vi "Process.vi"(8 "error in":errorcluster, 11 "SMO.UI.ByRefWithEvents":refnum<class "SMO.UI.ByRefWithEvents.lvclass">) -> (0 "error out":errorcluster, 3 "SMO.UI.ByRefWithEvents out":refnum<class "SMO.UI.ByRefWithEvents.lvclass">)   [LabVIEW 2013, in "SMO.UI.ByRefWithEvents.lvclass"]
doc: "---------------------------------------------------------------\nJKI State Machine Objects™\nhttp://jki.net/state-machine-objects/\nCopyright (C) 2005-2015, JKI <info@jki.net>\nALL RIGHTS RESERVEDJKI State Machine Objects (SMO) 1.0.0.5\nJKI - JKI\nCopyright (c) 2016, JKI"
uses:
  SMO.UI.ByRefWithEvents.lvclass
  <vilib>/JKI/JKI SMO/SMO/Typedefs/Parent Call--Enum.ctl
  <vilib>/JKI/JKI SMO/SMO.UI/SMO.UI.lvclass
  <vilib>/JKI/JKI SMO/SMO/SMO.lvclass
panel:
  out "Data":string
  # "For instructions on how to use the JKI State Machine Objects, examples and video tutorials, visit:\nhttp://jki.net/state-machine-objects/\n\nJKI State Machine Objects™\nhttp://jki.net/state-machine-objects/\nCopyright (C) 2005-2015, JKI <info@jki.net>\nALL RIGHTS RESERVED"
  # "SMO UI Template"
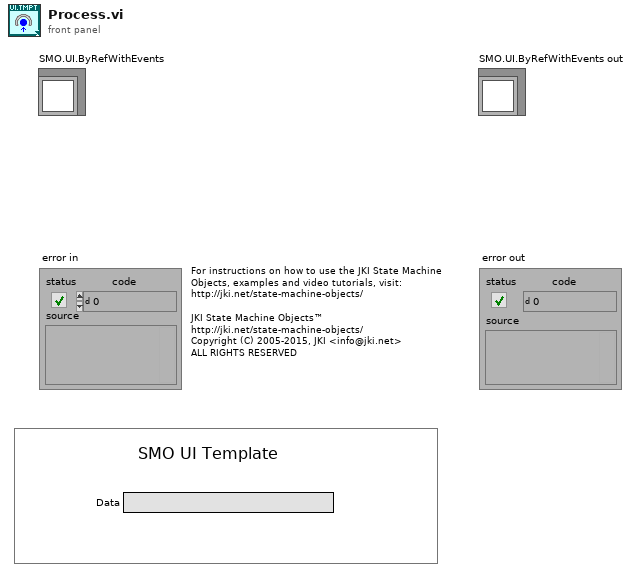
[diagram p1: front panel]
types:
  T1 = typedef "SMO.lvclass/Parent Call--Enum.ctl" = enum16{"Allows parent to run", "Does not request parent to run"}
  T2 = enum32{"invalid app kind", "Development System", "Run Time System", "Student Edition", "Embedded LabVIEW", "Evaluation", "Custom"}
  T3 = enum32{"Invalid", "Standard", "Closed", "Hidden", "Minimized", "Maximized"}
  T4 = cluster{"Core":cluster{"Current VI Reference":refnum<vi>, "Close Panel on Exit?":bool, "error":errorcluster}, "Self Reference":refnum<class "SMO.UI.ByRefWithEvents.lvclass">, "Your string data":string}
  T5 = cluster{"Current VI Reference":refnum<vi>, "Close Panel on Exit?":bool, "error":errorcluster}
  T6 = typedef "SMO.lvclass/Protected Events.ctl" = cluster{"StopProcesses":refnum<user-event>, "AbortProcesses":refnum<user-event>, "Config Changed":refnum<user-event>}
  T7 = typedef "SMO.UI.ByRefWithEvents.lvclass/ProtectedEvents--Cluster.ctl" = cluster{"API_Template":refnum<user-event>}
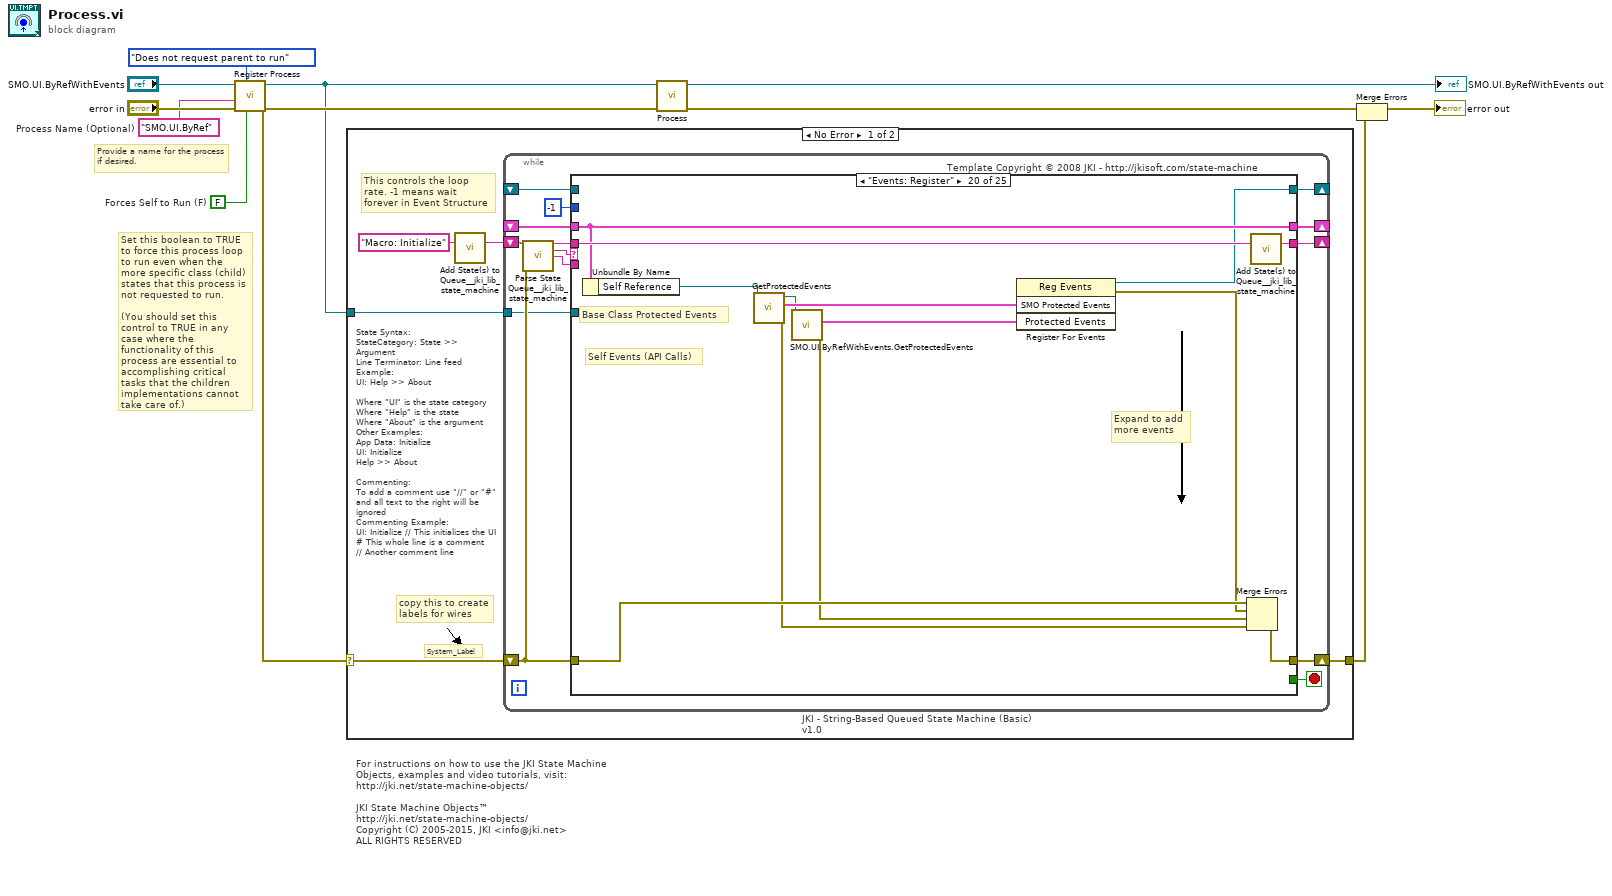
[diagram p0: block diagram]
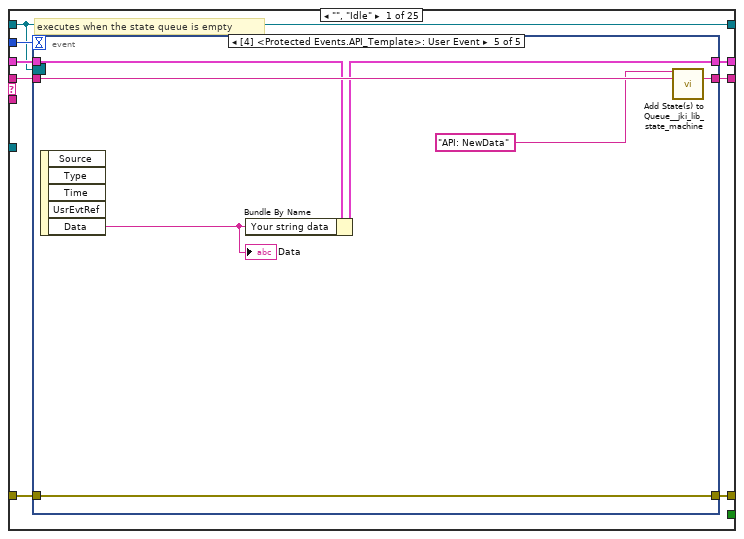
[diagram p2: hidden frame]
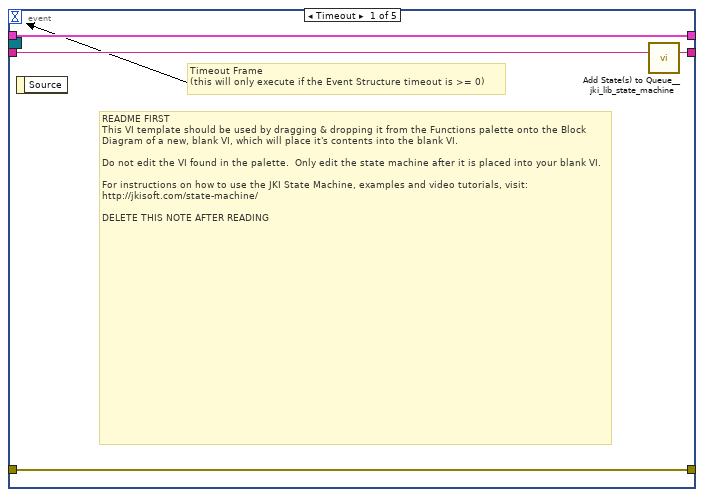
[diagram p3: hidden frame]
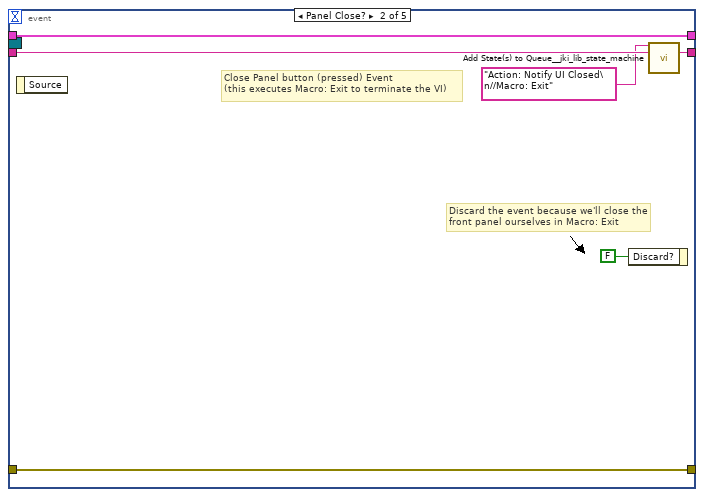
[diagram p4: hidden frame]
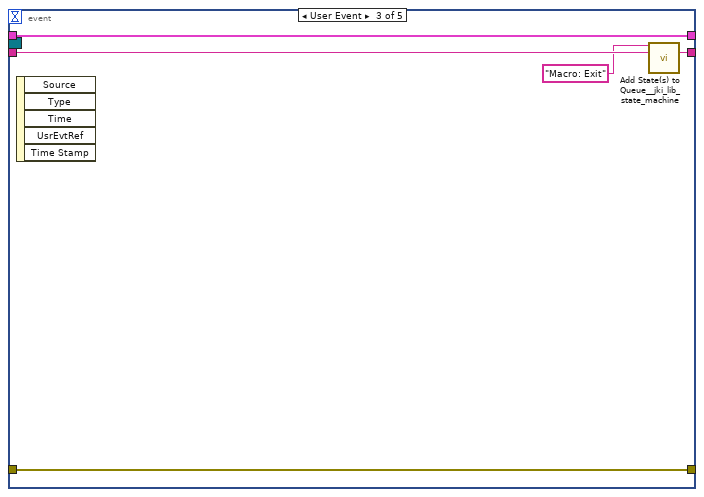
[diagram p5: hidden frame]
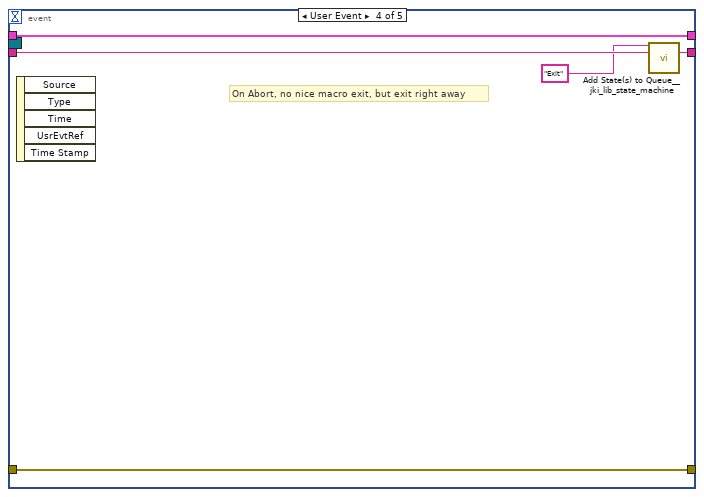
[diagram p6: hidden frame]
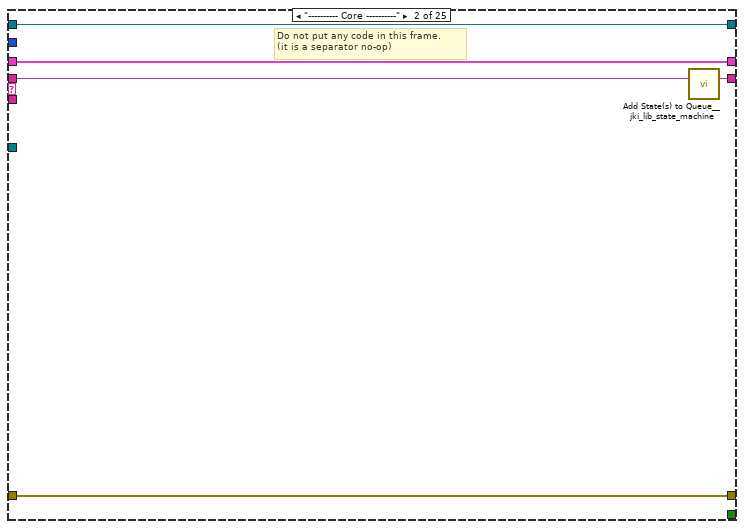
[diagram p7: hidden frame]
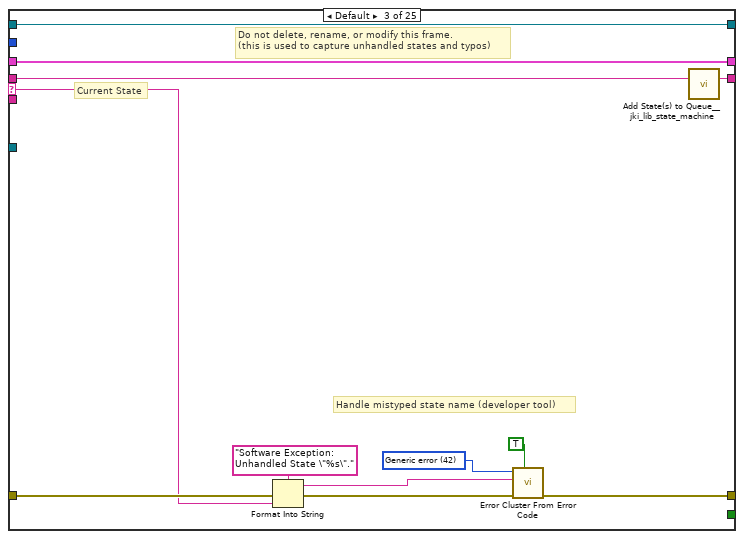
[diagram p8: hidden frame]
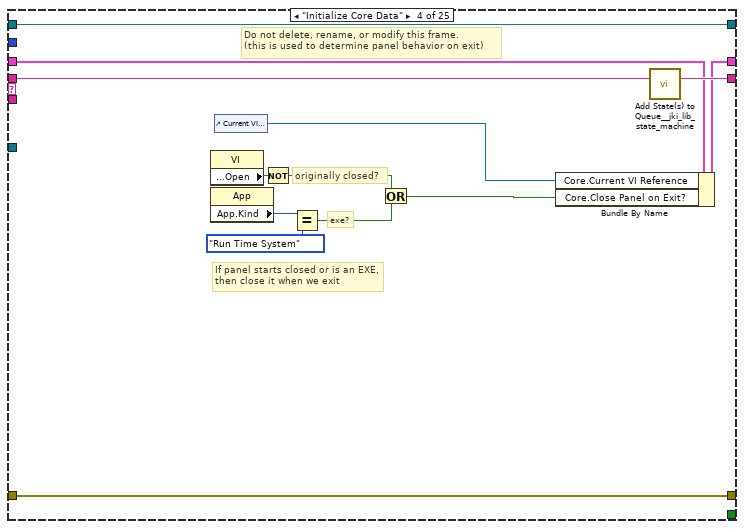
[diagram p9: hidden frame]
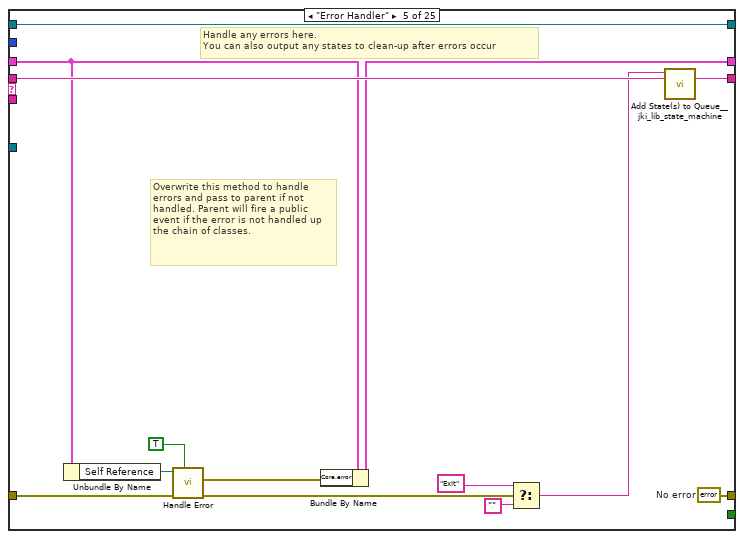
[diagram p10: hidden frame]
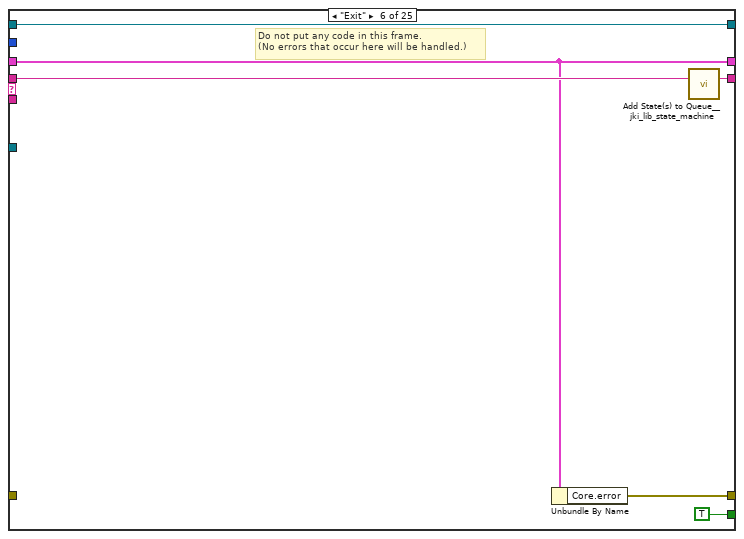
[diagram p11: hidden frame]
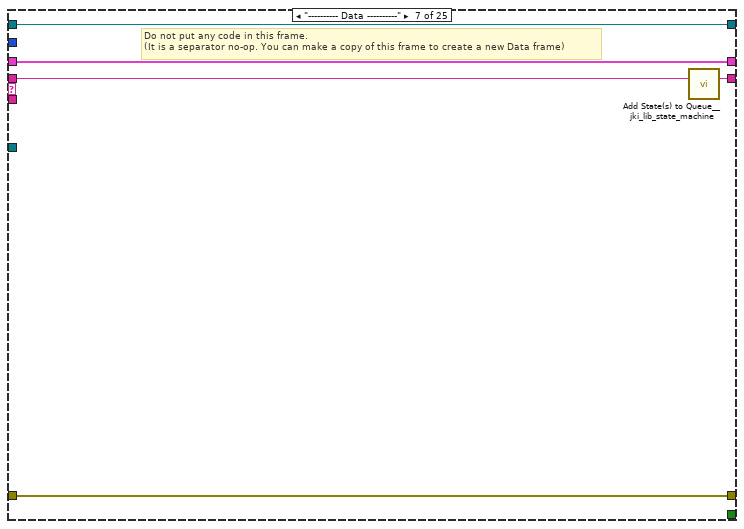
[diagram p12: hidden frame]
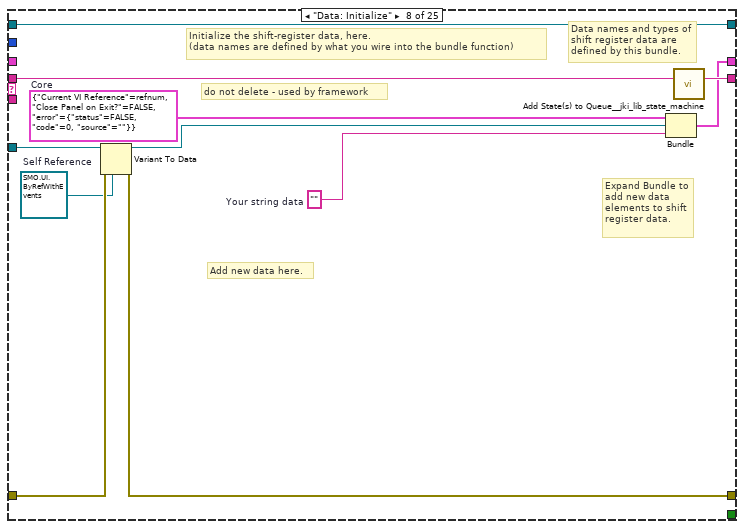
[diagram p13: hidden frame]
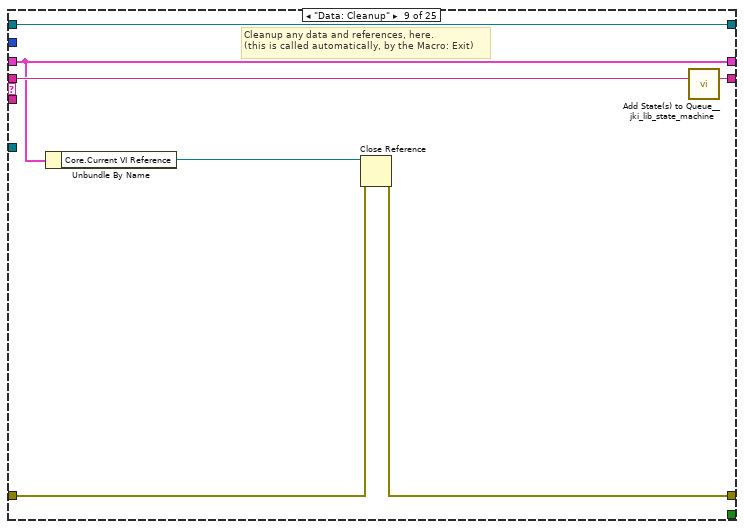
[diagram p14: hidden frame]
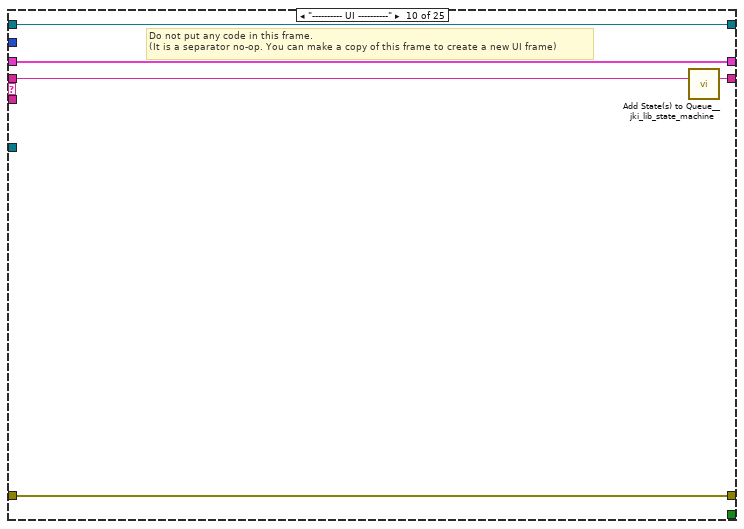
[diagram p15: hidden frame]
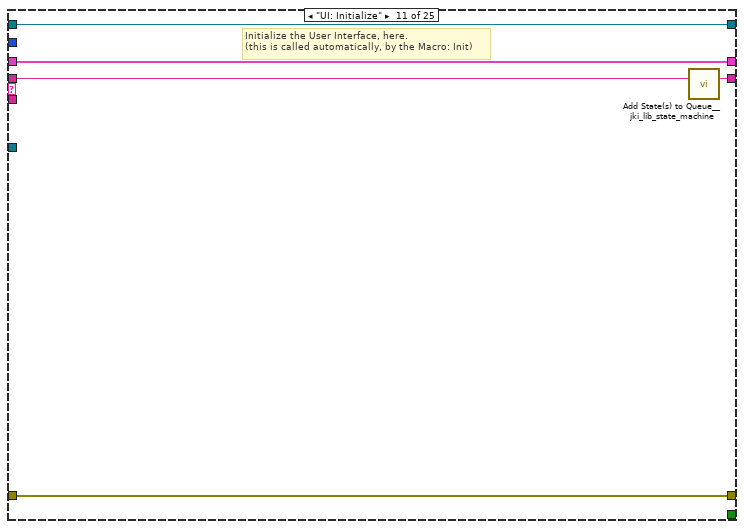
[diagram p16: hidden frame]
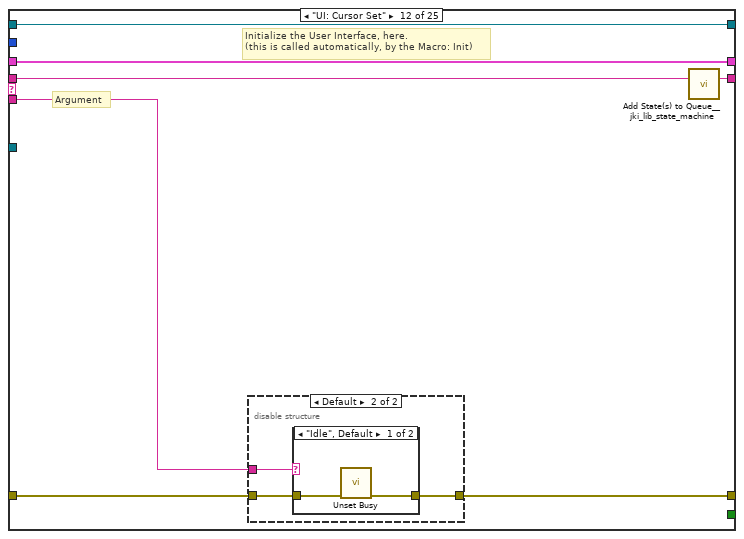
[diagram p17: hidden frame]
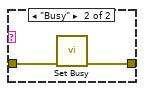
[diagram p19: hidden frame]
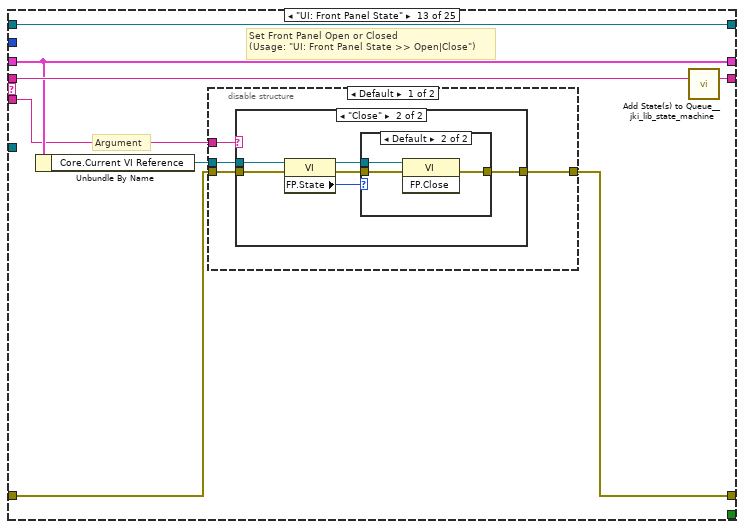
[diagram p20: hidden frame]
diagram:
  w2 = FALSE  # Forces Self to Run (F)
  w1 = "SMO.UI.ByRef"  # Process Name (Optional)
  # "Provide a name for the process\nif desired."
  # "Set this boolean to TRUE to force this process loop to run even when the more specific class (child) states that this process is not requested to run.\n\n(You should set this control to TRUE in any case where the functionality of this process are essential to accomplishing critical tasks that the children implementations cannot take care of.)"
  # "For instructions on how to use the JKI State Machine Objects, examples and video tutorials, visit:\nhttp://jki.net/state-machine-objects/\n\nJKI State Machine Objects™\nhttp://jki.net/state-machine-objects/\nCopyright (C) 2005-2015, JKI <info@jki.net>\nALL RIGHTS RESERVED"
  n1 = call <vilib>:"Register Process.vi"("Forces Self to Run (F)"=w2, "Parent Call"=Parent_Call--Enum."Does not request parent to run", "error in (no error)"="error in", "Process Name (optional)"=w1, "SMO"="SMO.UI.ByRefWithEvents") -> ("error out"=w8:errorcluster, "SMO out"=w7:refnum<class "SMO.UI.ByRefWithEvents.lvclass">)  [unwired: 5 in]
  n2 = case shown="No Error" w8 {
    selector: w8 -> [w13 w292]
    tunnel: w7 -> [w14 _]
    tunnel: [w12 w292] -> w4
    frame No Error {
      # "State Syntax:\nStateCategory: State >> Argument\nLine Terminator: Line feed\nExample:\nUI: Help >> About\n\nWhere \"UI\" is the state category\nWhere \"Help\" is the state\nWhere \"About\" is the argument\nOther Examples:\nApp Data: Initialize\nUI: Initialize\nHelp >> About\n\nCommenting:\nTo add a comment use \"//\" or \"#\" and all text to the right will be ignored\nCommenting Example:\nUI: Initialize // This initializes the UI\n# This whole line is a comment\n// Another comment line"
      # "copy this to create labels for wires"
      # "This controls the loop rate. -1 means wait forever in Event Structure"
      # "System_Label"
      n3 = call <vilib>:"Add State(s) to Queue__jki_lib_state_machine.vi"("State(s) in (\"\")"="Macro: Initialize") -> ("States Out"=w16:string)  [unwired: 14 in]
      n4 = while "JKI - String-Based Queued State Machine (Basic) v1.0" {
        shift-right: [w23] -> _
        shift-left: _ -> [w22]
        shift-right: [w26] -> w12
        shift-left: w13 -> [w20]
        shift-right: [w25] -> _
        shift-left: w16 -> [w27]
        tunnel: w14 -> [w19]
        shift-right: [w18] -> _
        shift-left: _ -> [w17]
        stop <- w24 stop-if-true
        # "Template Copyright © 2008 JKI - http://jkisoft.com/state-machine"
        n5 = call <vilib>:"Parse State Queue__jki_lib_state_machine.vi"("State Queue"=w27, "Error In (no error)"=w20) -> ("Remaining States"=w29:string, "Current State"=w30:string, "Arguments"=w28:string)  [unwired: 11 in]
        n6 = case shown="\"Events: Register\"" w30 {
          selector: w30 -> [_ _ w72 _ _ _ _ _ _ _ _ _ _ _ _ _ _ _ _ _ _ _ _ _ _]
          tunnel: w29 -> [w38 w70 w76 w95 w109 w115 w120 w131 w138 w143 w148 w155 w171 w203 w212 w226 w231 w242 w247 w260 w266 w271 w279 w284 w291]
          tunnel: w28 -> [_ _ _ _ _ _ _ _ _ _ _ w149 w165 _ _ _ _ _ _ _ _ _ _ _ _]
          tunnel: w22 -> [w36 w67 w74 w86 w98 w111 w117 _ w133 w140 w146 w153 w167 w200 w208 w217 w228 w239 w244 w258 w264 w269 w276 w282 w287]
          tunnel: [w35 w68 w78 w92 w100 w110 w118 w126 w134 w141 w145 w150 w168 w201 w210 w224 w229 w233 w245 w250 w262 w267 w273 w280 w285] -> w26
          tunnel: w20 -> [w34 w68 w77 w92 w105 _ w118 w127 w135 w141 w145 w151 w169 w201 w210 w224 w229 w234 w245 w252 w262 w267 w274 w280 w286]
          tunnel: [w37 w69 w75 w94 w108 w114 w119 w130 w137 w142 w147 w154 w170 w202 w211 w225 w230 w241 w246 w259 w265 w270 w278 w283 w290] -> w25
          tunnel: [_ _ _ _ _ TRUE _ _ _ _ _ _ _ _ _ _ _ _ _ _ _ _ _ _ _] -> w24
          tunnel: [w33 w67 w74 w93 w97 w111 w117 w129 w133 w140 w146 w153 w167 w200 w208 w217 w228 w239 w244 w258 w264 w269 w276 w282 w287] -> w23
          tunnel: -1 ("Timeout") -> [w32 _ _ _ _ _ _ _ _ _ _ _ _ _ _ _ _ _ _ _ _ _ _ _ _]
          tunnel: w19 -> [_ _ _ _ _ _ _ w124 _ _ _ _ _ _ _ _ _ _ _ _ _ _ _ _ _]
          tunnel: [w31 w66 w71 w83 w107 w112 w116 w122 w132 w139 w144 w152 w164 w199 w209 w218 w227 w240 w243 w257 w263 w268 w277 w281 w289] -> w18
          tunnel: w17 -> [w31 w66 w71 w83 w107 w112 w116 w122 w132 w139 w144 w152 w164 w199 w209 w218 w227 w240 w243 _ w263 w268 w277 w281 w289]
          frame "", "Idle" {
            # "executes when the state queue is empty"
            n7 = event shown="[4] <Protected Events.API_Template>: User Event" {
              selector: w31 -> [_ _ _ _ _]
              dyn-events: _ -> [_ _ _ _ _]
              timeout: w32 -> [_ _ _ _ _]
              tunnel: w38 -> [w42 w48 w53 w58 w65]
              tunnel: [w41 w47 w52 w57 w64] -> w37
              tunnel: w36 -> [w39 w44 w50 w55 w62]
              tunnel: [w40 w43 w51 w56 w63] -> w35
              tunnel: w34 -> [w40 w43 w51 w56 w63]
              tunnel: [w39 w44 w50 w55 w61] -> w33
              event Timeout {
                # "README FIRST\nThis VI template should be used by dragging & dropping it from the Functions palette onto the Block Diagram of a new, blank VI, which will place it's contents into the blank VI.\n\nDo not edit the VI found in the palette.  Only edit the state machine after it is placed into your blank VI.\n\nFor instructions on how to use the JKI State Machine, examples and video tutorials, visit:\nhttp://jkisoft.com/state-machine/\n\nDELETE THIS NOTE AFTER READING"
                # "Timeout Frame\n(this will only execute if the Event Structure timeout is >= 0)"
                n8 = event-data() -> ()  [unwired: 1 in, 1 out]
                n9 = call <vilib>:"Add State(s) to Queue__jki_lib_state_machine.vi"("State(s) in (\"\")"=w42) -> ("States Out"=w41:string)  [unwired: 14 in]
              }
              event Panel Close? {
                # "Discard the event because we'll close the front panel ourselves in Macro: Exit"
                # "Close Panel button (pressed) Event\n(this executes Macro: Exit to terminate the VI)"
                n10 = event-data() -> ()  [unwired: 1 in, 1 out]
                n11 = event-data("Discard?"=FALSE) -> ()  [unwired: 1 in, 1 out]
                n12 = call <vilib>:"Add State(s) to Queue__jki_lib_state_machine.vi"("State(s) in Front (\"\")"="Action: Notify UI Closed\n//Macro: Exit", "State(s) in (\"\")"=w48) -> ("States Out"=w47:string)  [unwired: 13 in]
              }
              event User Event {
                n13 = event-data() -> ()  [unwired: 1 in, 5 out]
                n14 = call <vilib>:"Add State(s) to Queue__jki_lib_state_machine.vi"("State(s) in Front (\"\")"="Macro: Exit", "State(s) in (\"\")"=w53) -> ("States Out"=w52:string)  [unwired: 13 in]
              }
              event User Event {
                # "On Abort, no nice macro exit, but exit right away"
                n15 = event-data() -> ()  [unwired: 1 in, 5 out]
                n16 = call <vilib>:"Add State(s) to Queue__jki_lib_state_machine.vi"("State(s) in Front (\"\")"="Exit", "State(s) in (\"\")"=w58) -> ("States Out"=w57:string)  [unwired: 13 in]
              }
              event User Event {
                n17 = event-data() -> ("Data"=w59:string)  [unwired: 1 in, 4 out]
                "Data" <- w59
                n18 = Bundle By Name(cluster=w62, "Your string data"=w59) -> (w61:T4)
                n19 = call <vilib>:"Add State(s) to Queue__jki_lib_state_machine.vi"("State(s) in Front (\"\")"="API: NewData", "State(s) in (\"\")"=w65) -> ("States Out"=w64:string)  [unwired: 13 in]
              }
            }
          }
          frame "---------- Core ----------" {
            # "Do not put any code in this frame.\n(it is a separator no-op)"
            n20 = call <vilib>:"Add State(s) to Queue__jki_lib_state_machine.vi"("State(s) in (\"\")"=w70) -> ("States Out"=w69:string)  [unwired: 14 in]
          }
          frame Default {
            w81 = 42 items=["No error", "Argument error", "Memory is full", "Out of zone", "End of file", "File already open", "Generic file I/O error", "File not found", "File permission error", "Disk is full", "Duplicate path", "Too many files open", "System feature not enabled", "Resource file not found", "Cannot add resource", "Resource not found", "Image not found", "Image memory error", "Pen does not exist", "Config type invalid", "Config token not found", "Config parse error", "Config memory error", "Bad external code format", "Bad external code offset", "External code not present", "Null window", "Destroy window error", "Null menu", "Print aborted", "Bad print record", "Print driver error", "Windows error during printing", "Memory error during printing", "Print dialog error", "Generic print error", "Invalid device refnum", "Device not found", "Device parameter error", "Device unit error", "Cannot open device", "Device call aborted", "Generic error", "Cancelled by user", "Object ID too low", "Object ID too high", "Object not in heap", "Unknown heap", "Unknown object (invalid DefProc)", "Unknown object (DefProc not in table)", "Message out of range", "Invalid (null) method", "Unknown message", "Manager call not supported", "Bad address", "Network operation in progress", "Network operation timed out", "Connection is busy", "Network attribute not supported", "Network error", "Address in use", "System out of memory", "Connection aborted", "Connection refused", "Not connected", "Already connected", "Connection closed", "Initialization error (interapplication manager)", "Bad occurrence", "Wait on unbound occurrence handler", "Occurrence queue overflow", "Datalog type conflict", "Unused", "Unrecognized type (interapplication manager)", "Memory corrupt", "Failed to make temporary DLL", "Old CIN version", "Drag socket not found", "Failed to load drop-object", "Failed to register OLE object", "Failed to release OLE object", "Format specifier type mismatch", "Unknown format specifier", "Too few format specifiers", "Too many format specifiers", "Scan failed", "Newer CIN version", "Error converting to variant", "Runtime menu error", "Password tampered", "Variant attribute not found", "Incompatible variant data type", "Event data is not available", "Event Store is not present", "Occurrence is not found", "Event Queue is not created", "Event info is not available", "Refnum passed is NULL", "Error retrieving Class GUID", "Error retrieving CoClass GUID", "Error retrieving TypeLib GUID.", "Bad built application magic bytes.", "Specific driver is different from the specific driver associated with the Logical Name.", "There is no session opened to the class driver.", "Max Error", "MAX - Error with config objects", "MAX - Error loading configuration", "MAX - Group not supported"]
            # "Current State"
            # "Do not delete, rename, or modify this frame.\n(this is used to capture unhandled states and typos)"
            # "Handle mistyped state name (developer tool)"
            n21 = Format Into String(format string="Software Exception: Unhandled State \"%s\"." ("message"), error in=w77, w72) -> (resulting string=w80:string, error out=w79:errorcluster)  [unwired: 1 in]
            n22 = call <vilib>:"Error Cluster From Error Code.vi"("show call chain? (False)"=TRUE, "error in (no error)"=w79, "error message (\"\")"=w80, "error code (0)"=w81) -> ("error out"=w78:errorcluster)  [unwired: 5 in]
            n23 = call <vilib>:"Add State(s) to Queue__jki_lib_state_machine.vi"("State(s) in (\"\")"=w76) -> ("States Out"=w75:string)  [unwired: 14 in]
          }
          frame "Initialize Core Data" {
            # "Do not delete, rename, or modify this frame.\n(this is used to determine panel behavior on exit)"
            # "originally closed?"
            # "exe?"
            # "If panel starts closed or is an EXE, then close it when we exit"
            n24 = property class="VI"() -> ("Front Panel.Open"=w91:bool)  [unwired: 2 in, 2 out]
            n25 = property class="App"() -> ("App.Kind"=w90:T2)  [unwired: 2 in, 2 out]
            n26 = control-ref of="Current VI Reference"() -> (w84:refnum<vi>)
            n27 = Not(x=w91) -> (.not. x?=w88:bool)
            n28 = Equal?(x=w90, y=T2."Run Time System" ("Application:Kind")) -> (x = y?=w87:bool)
            n29 = Or(x=w88, y=w87) -> (x .or. y?=w85:bool)
            n30 = Bundle By Name(cluster=w86, "Core.Current VI Reference"=w84, "Core.Close Panel on Exit?"=w85) -> (w93:T4)
            n31 = call <vilib>:"Add State(s) to Queue__jki_lib_state_machine.vi"("State(s) in (\"\")"=w95) -> ("States Out"=w94:string)  [unwired: 14 in]
          }
          frame "Error Handler" {
            w100 = errorcluster {"status"=FALSE, "code"=0, "source"=""}  # No error
            # "Overwrite this method to handle errors and pass to parent if not handled. Parent will fire a public event if the error is not handled up the chain of classes."
            # "Handle any errors here.\nYou can also output any states to clean-up after errors occur"
            n32 = Unbundle By Name(w98) -> ("Self Reference"=w106:refnum<class "SMO.UI.ByRefWithEvents.lvclass">)
            n33 = call-dynamic "Handle Error.vi"("Stop on Unhandled Error (T)"=TRUE, "error in"=w105, "SMO"=w106) -> ("handling error"=w101:errorcluster, "Unhandled error"=w99:errorcluster)  [unwired: 6 in, 1 out]
            n34 = Bundle By Name(cluster=w98, "Core.error"=w99) -> (w97:T4)
            n35 = Select(t="Exit", s=w101, f="") -> (s? t:f=w102:string)
            n36 = call <vilib>:"Add State(s) to Queue__jki_lib_state_machine.vi"("State(s) in Front (\"\")"=w102, "State(s) in (\"\")"=w109) -> ("States Out"=w108:string)  [unwired: 13 in]
          }
          frame "Exit" {
            # "Do not put any code in this frame.\n(No errors that occur here will be handled.)"
            n37 = Unbundle By Name(w111) -> ("Core.error"=w110:errorcluster)
            n38 = call <vilib>:"Add State(s) to Queue__jki_lib_state_machine.vi"("State(s) in (\"\")"=w115) -> ("States Out"=w114:string)  [unwired: 14 in]
          }
          frame "---------- Data ----------" {
            # "Do not put any code in this frame.\n(It is a separator no-op. You can make a copy of this frame to create a new Data frame)"
            n39 = call <vilib>:"Add State(s) to Queue__jki_lib_state_machine.vi"("State(s) in (\"\")"=w120) -> ("States Out"=w119:string)  [unwired: 14 in]
          }
          frame "Data: Initialize" {
            w121 = T5 {"Current VI Reference"=refnum, "Close Panel on Exit?"=FALSE, "error"={"status"=FALSE, "code"=0, "source"=""}}  # Core
            w125 = refnum<class "SMO.UI.ByRefWithEvents.lvclass"> refnum  # Self Reference
            w128 = ""  # Your string data
            # "do not delete - used by framework"
            # "Expand Bundle to add new data elements to shift register data."
            # "Add new data here."
            # "Data names and types of shift register data are defined by this bundle."
            # "Initialize the shift-register data, here.\n(data names are defined by what you wire into the bundle function)"
            n40 = Variant To Data(error in=w127, type=w125, Variant=w124) -> (data=w123:refnum<class "SMO.UI.ByRefWithEvents.lvclass">, error out=w126:errorcluster)
            n41 = Bundle("Core"=w121, "Self Reference"=w123, "Your string data"=w128) -> (w129:T4)  [unwired: 1 in]
            n42 = call <vilib>:"Add State(s) to Queue__jki_lib_state_machine.vi"("State(s) in (\"\")"=w131) -> ("States Out"=w130:string)  [unwired: 14 in]
          }
          frame "Data: Cleanup" {
            # "Cleanup any data and references, here.\n(this is called automatically, by the Macro: Exit)"
            n43 = Unbundle By Name(w133) -> ("Core.Current VI Reference"=w136:refnum<vi>)
            n44 = Close Reference(reference=w136, error in (no error)=w135) -> (error out=w134:errorcluster)
            n45 = call <vilib>:"Add State(s) to Queue__jki_lib_state_machine.vi"("State(s) in (\"\")"=w138) -> ("States Out"=w137:string)  [unwired: 14 in]
          }
          frame "---------- UI ----------" {
            # "Do not put any code in this frame.\n(It is a separator no-op. You can make a copy of this frame to create a new UI frame)"
            n46 = call <vilib>:"Add State(s) to Queue__jki_lib_state_machine.vi"("State(s) in (\"\")"=w143) -> ("States Out"=w142:string)  [unwired: 14 in]
          }
          frame "UI: Initialize" {
            # "Initialize the User Interface, here.\n(this is called automatically, by the Macro: Init)"
            n47 = call <vilib>:"Add State(s) to Queue__jki_lib_state_machine.vi"("State(s) in (\"\")"=w148) -> ("States Out"=w147:string)  [unwired: 14 in]
          }
          frame "UI: Cursor Set" {
            # "Argument"
            # "Initialize the User Interface, here.\n(this is called automatically, by the Macro: Init)"
            n48 = disable-structure shown="Default" {
              disable-tunnel: w151 -> [w156 w159]
              disable-tunnel: [w156 w158] -> w150
              disable-tunnel: w149 -> [_ w157]
              frame condition #0 {
              }
              frame condition #1 (active) {
                n49 = case shown="\"Idle\", Default" w157 {
                  tunnel: w159 -> [w161 w163]
                  tunnel: [w160 w162] -> w158
                  frame "Idle", Default {
                    n50 = call <vilib>:"Unset Busy.vi"("error in (no error)"=w161) -> ("error out"=w160:errorcluster)  [unwired: 10 in]
                  }
                  frame "Busy" {
                    n51 = call <vilib>:"Set Busy.vi"("error in (no error)"=w163) -> ("error out"=w162:errorcluster)  [unwired: 9 in, 1 out]
                  }
                }
              }
            }
            n52 = call <vilib>:"Add State(s) to Queue__jki_lib_state_machine.vi"("State(s) in (\"\")"=w155) -> ("States Out"=w154:string)  [unwired: 14 in]
          }
          frame "UI: Front Panel State" {
            # "Argument"
            # "Set Front Panel Open or Closed\n(Usage: \"UI: Front Panel State >> Open|Close\")"
            n53 = Unbundle By Name(w167) -> ("Core.Current VI Reference"=w166:refnum<vi>)
            n54 = disable-structure shown="Default" {
              disable-tunnel: w169 -> [w175 w198]
              disable-tunnel: [w174 w198] -> w168
              disable-tunnel: w166 -> [w173 _]
              disable-tunnel: w165 -> [w172 _]
              frame condition #0 (active) {
                n55 = case shown="\"Close\"" w172 {
                  tunnel: w175 -> [w179 w192]
                  tunnel: [w181 w193] -> w174
                  tunnel: w173 -> [w180 w190]
                  frame "Open", Default {
                    n56 = property class="VI"(reference=w180, error in=w179) -> (reference out=w177:refnum<vi>, error out=w178:errorcluster, "FP.State"=w176:T3)
                    n57 = case shown="\"Closed\"" w176 {
                      tunnel: [w184 w187] -> w181
                      tunnel: w178 -> [w183 w187]
                      tunnel: w177 -> [w182 _]
                      frame "Closed" {
                        n58 = invoke class="VI" method="FP.Open"(reference=w182, error in=w183, "Activate"=TRUE, "State"=T3."Standard") -> (error out=w184:errorcluster)  [unwired: 1 in, 4 out]
                      }
                      frame Default {
                      }
                    }
                  }
                  frame "Close" {
                    n59 = property class="VI"(reference=w190, error in=w192) -> (reference out=w189:refnum<vi>, error out=w191:errorcluster, "FP.State"=w188:T3)
                    n60 = case shown="Default" w188 {
                      tunnel: [w194 w197] -> w193
                      tunnel: w191 -> [w194 w196]
                      tunnel: w189 -> [_ w195]
                      frame "Invalid", "Closed" {
                      }
                      frame Default {
                        n61 = invoke class="VI" method="FP.Close"(reference=w195, error in=w196) -> (error out=w197:errorcluster)  [unwired: 1 in, 2 out]
                      }
                    }
                  }
                }
              }
              frame condition #1 {
              }
            }
            n62 = call <vilib>:"Add State(s) to Queue__jki_lib_state_machine.vi"("State(s) in (\"\")"=w171) -> ("States Out"=w170:string)  [unwired: 14 in]
          }
          frame "---------- Macro ----------" {
            # "Do not put any code in this frame.\n(It is a separator no-op. You can make a copy of this frame to create a new Macro frame)"
            n63 = call <vilib>:"Add State(s) to Queue__jki_lib_state_machine.vi"("State(s) in (\"\")"=w203) -> ("States Out"=w202:string)  [unwired: 14 in]
          }
          frame "Macro: Initialize" {
            w206 = "UI: Initialize\n//UI: Front Panel State >> Open"  # UI: Initialize //UI: Front Panel State >> Open
            # "Initialization Macro\n(This is called once, when the VI starts)"
            n64 = call <vilib>:"Add State(s) to Queue__jki_lib_state_machine.vi"("State(s) in Front (\"\")"="Data: Initialize\nInitialize Core Data\nEvents: Register", "State(s) in (\"\")"="Process: Sync", "State(s) at Back (\"\")"=w206) -> ("States Out"=w205:string)  [unwired: 12 in]
            n65 = call <vilib>:"Add State(s) to Queue__jki_lib_state_machine.vi"("State(s) in Front (\"\")"=w205, "State(s) in (\"\")"=w212) -> ("States Out"=w211:string)  [unwired: 13 in]
          }
          frame "Macro: Exit" {
            # "Exit Macro\n(This is called once, when the VI exits)"
            n66 = Unbundle By Name(w217) -> ("Core.Close Panel on Exit?"=w223:bool)
            n67 = Select(t="//UI: Front Panel State >> Close", s=w223, f="") -> (s? t:f=w220:string)
            n68 = call <vilib>:"Add State(s) to Queue__jki_lib_state_machine.vi"("State(s) in Front (\"\")"="Data: Cleanup\nEvents: Unregister", "State(s) in (\"\")"="Process: Sync", "State(s) at Back (\"\")"="Exit") -> ("States Out"=w214:string)  [unwired: 12 in]
            n69 = call <vilib>:"Add State(s) to Queue__jki_lib_state_machine.vi"("State(s) in (\"\")"=w220, "State(s) at Back (\"\")"=w214) -> ("States Out"=w219:string)  [unwired: 13 in]
            n70 = call <vilib>:"Add State(s) to Queue__jki_lib_state_machine.vi"("State(s) in Front (\"\")"=w219, "State(s) in (\"\")"=w226) -> ("States Out"=w225:string)  [unwired: 13 in]
          }
          frame "---------- Process ----------" {
            # "Template Separator\n(You can make a copy of, or modify, this frame)"
            n71 = call <vilib>:"Add State(s) to Queue__jki_lib_state_machine.vi"("State(s) in (\"\")"=w231) -> ("States Out"=w230:string)  [unwired: 14 in]
          }
          frame "Process: Sync" {
            n72 = Unbundle By Name(w239) -> ("Self Reference"=w235:refnum<class "SMO.UI.ByRefWithEvents.lvclass">)
            n73 = call <vilib>:"WaitOnProcessSync.vi"("error in (no error)"=w234, "SMO"=w235) -> ("error out"=w233:errorcluster, "Don't run?"=w238:bool)  [unwired: 7 in, 1 out]
            n74 = Select(t="Data: Cleanup\nEvents: Unregister\nExit", s=w238, f="") -> (s? t:f=w232:string)
            n75 = call <vilib>:"Add State(s) to Queue__jki_lib_state_machine.vi"("State(s) in Front (\"\")"=w232, "State(s) in (\"\")"=w242) -> ("States Out"=w241:string)  [unwired: 13 in]
          }
          frame "---------- Events ----------" {
            # "Template Separator\n(You can make a copy of, or modify, this frame)"
            n76 = call <vilib>:"Add State(s) to Queue__jki_lib_state_machine.vi"("State(s) in (\"\")"=w247) -> ("States Out"=w246:string)  [unwired: 14 in]
          }
          frame "Events: Register" {
            # "Expand to add\nmore events"
            # "Self Events (API Calls)"
            # "Base Class Protected Events"
            n77 = Unbundle By Name(w258) -> ("Self Reference"=w253:refnum<class "SMO.UI.ByRefWithEvents.lvclass">)
            n78 = call <vilib>:"GetProtectedEvents.vi"("SMO"=w253) -> ("error out"=w248:errorcluster, "SMO Protected Events"=w256:T6, "SMO out"=w255:refnum<class "SMO.UI.ByRefWithEvents.lvclass">)  [unwired: 8 in]
            n79 = call "SMO.UI.ByRefWithEvents.GetProtectedEvents.vi"("SMO.UI.ByRefWithEvents"=w255) -> ("error out"=w249:errorcluster, "Protected Events"=w254:T7)  [unwired: 8 in, 1 out]
            n80 = register-events(w256, w254) -> (reference out=w257:refnum<event-registration>, error out=w251:errorcluster)  [unwired: 2 in]
            n81 = Merge Errors(w252, w251, w249, w248) -> (w250:errorcluster)
            n82 = call <vilib>:"Add State(s) to Queue__jki_lib_state_machine.vi"("State(s) in (\"\")"=w260) -> ("States Out"=w259:string)  [unwired: 14 in]
          }
          frame "Events: Unregister" {
            n83 = Unregister For Events(event registration refnum=w263, error in=w262) -> (error out=w261:errorcluster)
            n84 = call <vilib>:"Clear Errors.vi"("error in (no error)"=w261) -> ()  [unwired: 6 in, 1 out]
            n85 = call <vilib>:"Add State(s) to Queue__jki_lib_state_machine.vi"("State(s) in (\"\")"=w266) -> ("States Out"=w265:string)  [unwired: 14 in]
          }
          frame "---------- API ----------" {
            n86 = call <vilib>:"Add State(s) to Queue__jki_lib_state_machine.vi"("State(s) in (\"\")"=w271) -> ("States Out"=w270:string)  [unwired: 14 in]
          }
          frame "API: NewData" {
            n87 = Unbundle By Name(w276) -> ("Self Reference"=w272:refnum<class "SMO.UI.ByRefWithEvents.lvclass">, "Your string data"=w275:string)
            n88 = call "SMO.UI.ByRefWithEvents.SetData.vi"("error in (no error)"=w274, "Data In"=w275, "SMO.UI.ByRefWithEvents"=w272) -> ("error out"=w273:errorcluster)  [unwired: 7 in, 1 out]
            n89 = call <vilib>:"Add State(s) to Queue__jki_lib_state_machine.vi"("State(s) in (\"\")"=w279) -> ("States Out"=w278:string)  [unwired: 14 in]
          }
          frame "---------- Action ----------" {
            n90 = call <vilib>:"Add State(s) to Queue__jki_lib_state_machine.vi"("State(s) in (\"\")"=w284) -> ("States Out"=w283:string)  [unwired: 14 in]
          }
          frame "Action: Notify UI Closed" {
            # "Notify that the UI has been closed"
            n91 = Unbundle By Name(w287) -> ("Self Reference"=w288:refnum<class "SMO.UI.ByRefWithEvents.lvclass">)
            n92 = call <vilib>:"Hide.vi"("error in (no error)"=w286, "SMO.UI"=w288) -> ("error out"=w285:errorcluster)  [unwired: 8 in, 1 out]
            n93 = call <vilib>:"Add State(s) to Queue__jki_lib_state_machine.vi"("State(s) in (\"\")"=w291) -> ("States Out"=w290:string)  [unwired: 14 in]
          }
        }
      }
    }
    frame Error {
    }
  }
  n94 = call-parent "Process.vi"("error in (no error)"=w8, "SMO.UI"=w7) -> ("error out"=w5:errorcluster, "SMO.UI out"=→"SMO.UI.ByRefWithEvents out":refnum<class "SMO.UI.ByRefWithEvents.lvclass">)  [unwired: 8 in]
  n95 = Merge Errors(w5, w4) -> (→"error out":errorcluster)
